vi "TCP-invoke-error.vi"(6 "Return-code":T1 items=["Success"=0, "Bad Command"=8, "Bad Arg"=9, "No Files Found"=100, "No Drive"=101, "Not In Host Control"=106, "Wrong Host Type"=107, "Error Job Busy"=108, "Error Software"=110, "Cannot Create Port"=206, "Cannot Open Port"=207, "Port Not Open"=208, "Port Timeout"=209, "Wrong Port Number"=210], 8 "error in (no error)":errorcluster, 9 "Overwrite?":bool, 10 "Additional message":string) -> (0 "error out":errorcluster)   [LabVIEW 2013, in "SLMControl.lvlib" / "SM1000.lvclass"]
uses:
  SM1000.lvclass
  TCP-return-codes.ctl
  <vilib>/Utility/error.llb/DialogType.ctl
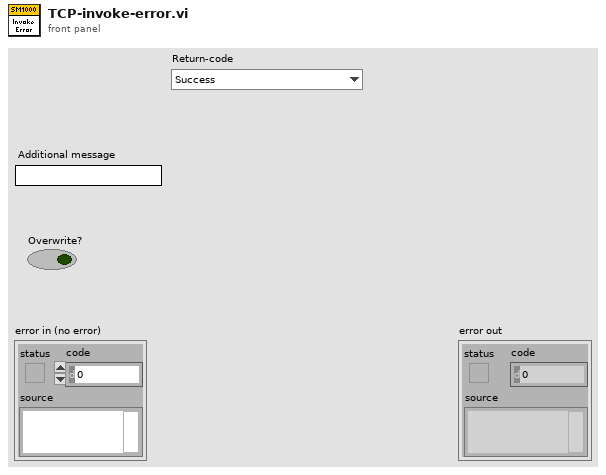
[diagram p1: front panel]
types:
  T1 = typedef "SLMControl.lvlib/SM1000.lvclass/TCP-return-codes.ctl" = i32
  T2 = typedef "DialogType.ctl" = u16
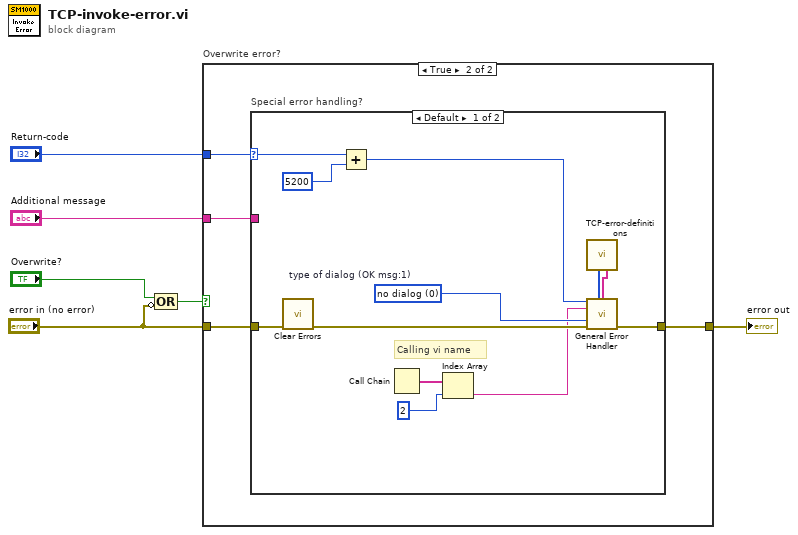
[diagram p0: block diagram]
diagram:
  n1 = Compound Arithmetic op=OR("Overwrite?", invert "error in (no error)") -> (w2:bool)
  n2 = case "Overwrite error?" shown="True" w2 {
    tunnel: [w7 w8] -> w6
    tunnel: "Return-code" -> [_ w11]
    tunnel: "Additional message" -> [_ w10]
    tunnel: "error in (no error)" -> [w7 w9]
    frame False {
    }
    frame True {
      n3 = case "Special error handling?" shown="Default" w11 {
        selector: w11 -> [w19 _]
        tunnel: [w22 w24] -> w8
        tunnel: w10 -> [_ _]
        tunnel: w9 -> [w23 w24]
        frame Default {
          w18 = T2 0 items=["no dialog", "OK message", "continue or stop message", "OK message + warnings", "continue/stop + warnings"]  # type of dialog (OK msg:1)
          # "Calling vi name"
          n4 = call <vilib>:"Clear Errors.vi"("error in (no error)"=w23) -> ("error out"=w17:errorcluster)  [unwired: 6 in]
          n5 = Add(x=w19, y=5200) -> (x+y=w21:T1)
          n6 = Call Chain() -> (call chain=w16:string[])
          n7 = Index Array(array=w16, index=2) -> (element=w14:string)
          n8 = call "TCP-error-definitions.vi"() -> ("Descriptions"=w12:string[], "Error codes"=w13:i32[])  [unwired: 10 in]
          n9 = call <vilib>:"General Error Handler.vi"("[error code] (0)"=w21, "[user-defined codes]"=w13, "[user-defined descriptions]"=w12, "[error source] (\" \")"=w14, "type of dialog (OK msg:1)"=w18, "error in (no error)"=w17) -> ("error out"=w22:errorcluster)  [unwired: 5 in, 4 out]
        }
        frame 0 {
          # "No error."
        }
      }
    }
  }
  "error out" <- w6
